vi "ColorizeREPL.vi"(0 "Refs":T1, 2 "FileName":string="Colors.txt", 4 "Add Spaces?":bool) -> (8 "Value":string)   [LabVIEW 2020]
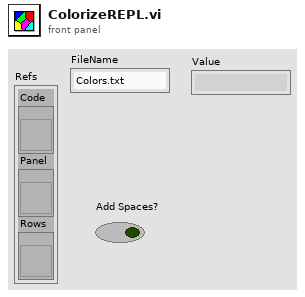
[diagram p1: front panel]
types:
  T1 = cluster{"Code":refnum<vi>, "Panel":refnum<vi>, "Rows":refnum<vi>}
  T2 = cluster{"Quote":u32, "Comment":u32, "Python":u32, "Text":u32, "Triple Quote":u32, "function":u32, "Line numbers":u32, "REPL Err":u32, "REPL Text":u32, "Text Bkgd":u32, "REPL Bkgd":u32}
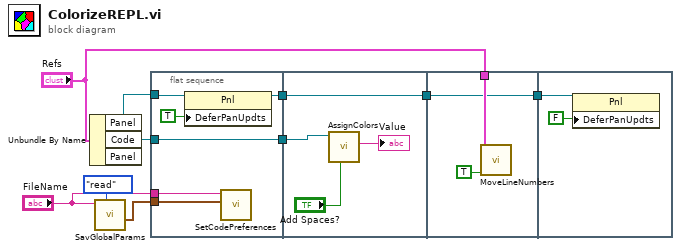
[diagram p0: block diagram]
diagram:
  n1 = Unbundle By Name("Refs") -> ("Panel"=w7:refnum<vi>, "Code"=w10:refnum<vi>)  [unwired: 1 out]
  n2 = call "SavGlobalParams.vi"("Task"=enum16{"read", "write"}."read", "FileName"="FileName") -> ("Colors Out"=w2:T2)  [unwired: 9 in]
  n3 = flat-sequence {
    tunnel: w10 -> [w16]
    tunnel: [w16] -> w8
    tunnel: w7 -> [w15]
    tunnel: [w13] -> w4
    tunnel: w2 -> [w12]
    tunnel: "FileName" -> [w11]
    tunnel: w8 -> [w19]
    tunnel: [w18] -> w5
    tunnel: w4 -> [w18]
    tunnel: "Refs" -> [w22]
    tunnel: [w21] -> w6
    tunnel: w5 -> [w21]
    tunnel: w6 -> [w24]
    frame #0 {
      n4 = property class="Pnl"(reference=w15, "DeferPanUpdts"=TRUE ("Defer Panel Updates")) -> (reference out=w13:refnum<vi>)  [unwired: 1 in, 1 out]
      n5 = call "SetCodePreferences.vi"("Color choices"=w12, "PrefFile"=w11) -> ()  [unwired: 10 in]
    }
    frame #1 {
      n6 = call "AssignColors.vi"("Add Spaces?"="Add Spaces?", "Code"=w19) -> ("Value"=→"Value":string)  [unwired: 9 in]
    }
    frame #2 {
      n7 = call "MoveLineNumbers.vi"("Force?"=TRUE, "Refs"=w22) -> ()  [unwired: 10 in]
    }
    frame #3 {
      n8 = property class="Pnl"(reference=w24, "DeferPanUpdts"=FALSE ("Defer Panel Updates")) -> ()  [unwired: 1 in, 2 out]
    }
  }
